vi "深国电程序控制(new).vi"(11 "槽位号":i16=1) -> ()   [LabVIEW 2012]
doc: "打开板卡操作，输出板卡句柄！当有多个板卡时，根据板卡索引号打开不同板卡！\n如果同时使用一块板卡的多种功能，可将输出句柄连接到不同的功能任务中。\n此VI是创建所有任务的前提！"
uses:
  P3060NEW/_SubVI/dll/P3060.dll
panel:
  in  "error IO":errorcluster
  out "波形图":i32[](graph)
  in  "read":bool caption="确定按钮"
  in  "LED¿ØÖÆû":bool
  in  "FPGA-Bit文件路径":path
  in  "加载程序":bool caption="确定按钮"
  in  "取消按钮":bool
  out "error out":errorcluster caption="错误警告"
  # "c"
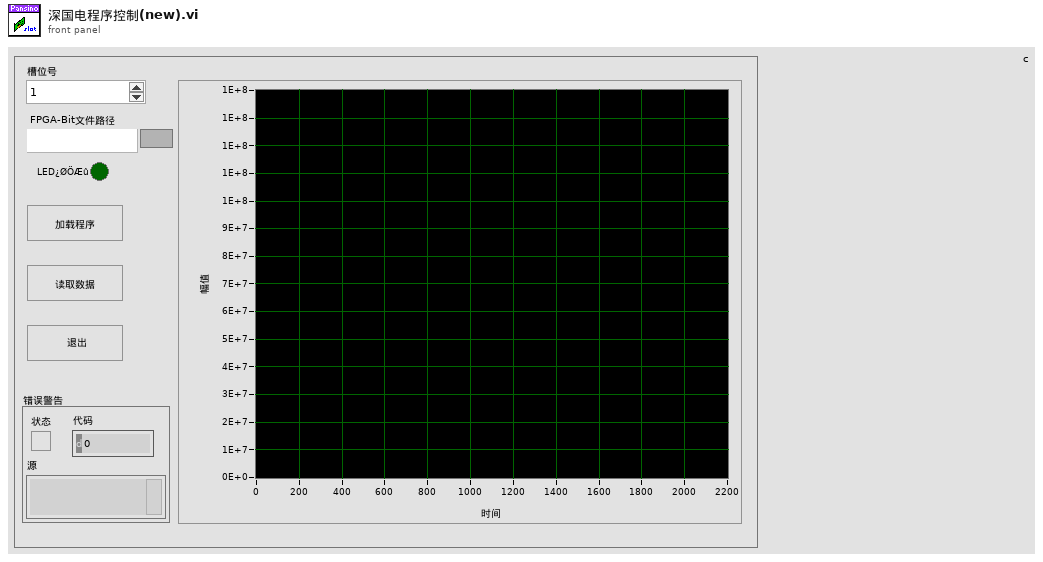
[diagram p1: front panel]
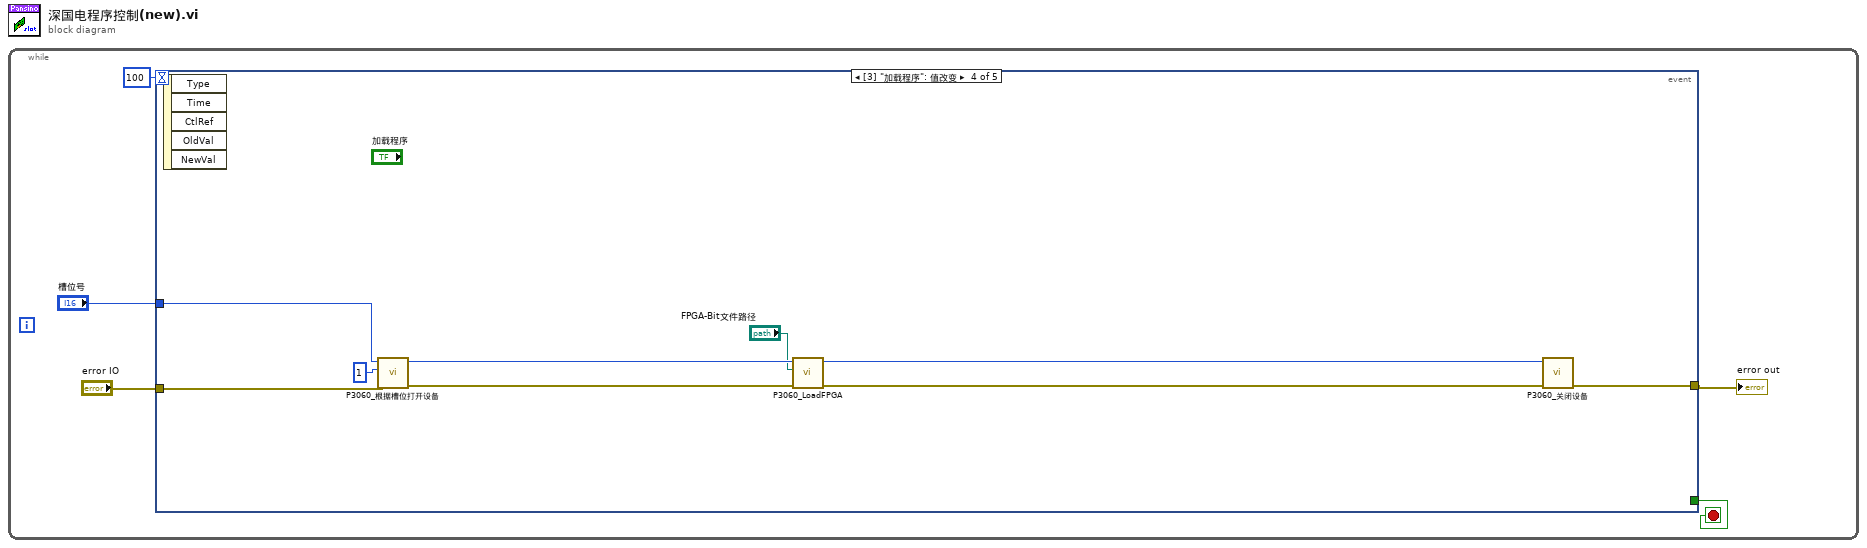
[diagram p0: block diagram]
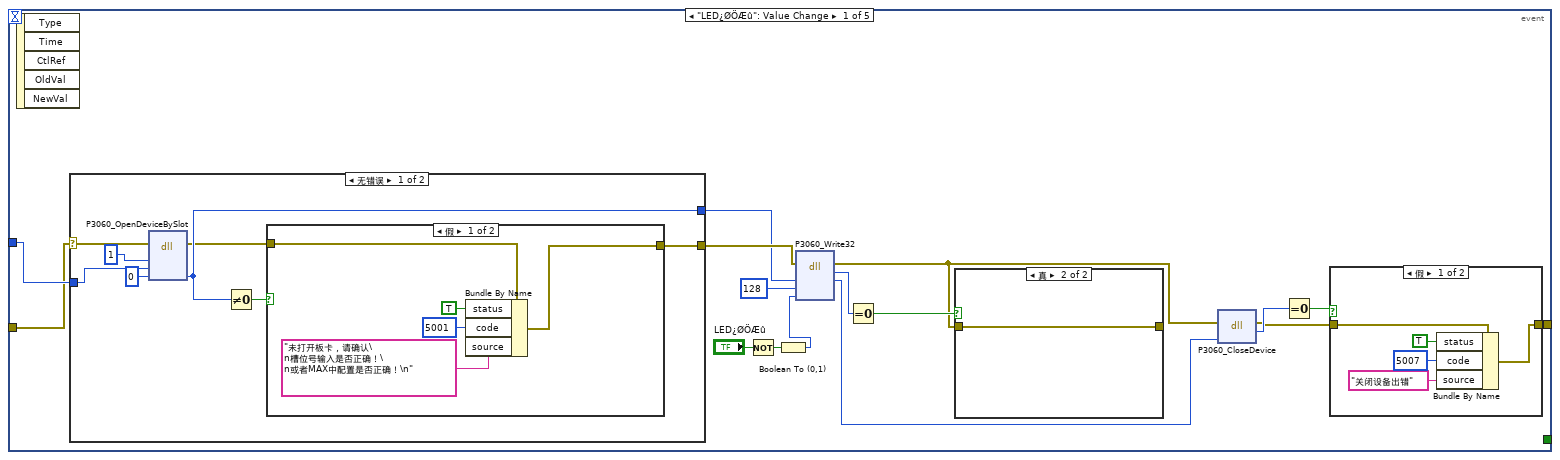
[diagram p2: hidden frame]
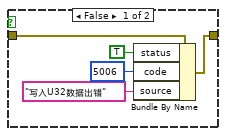
[diagram p3: hidden frame]
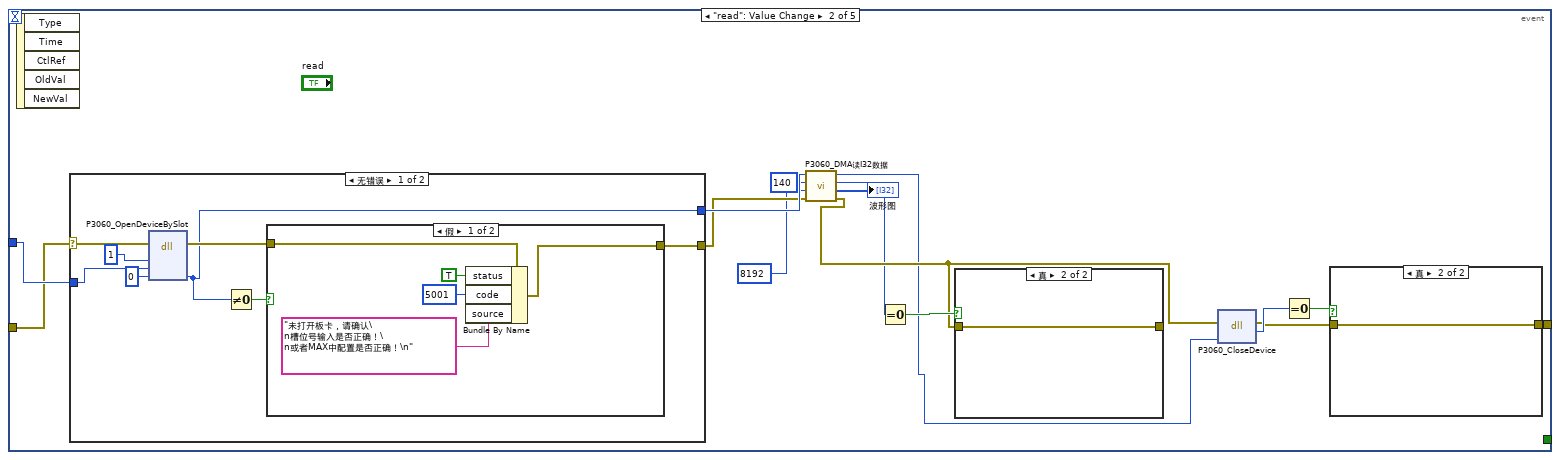
[diagram p7: hidden frame]
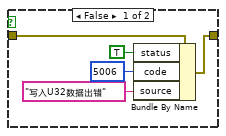
[diagram p8: hidden frame]
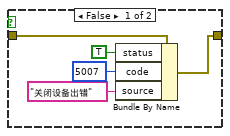
[diagram p9: hidden frame]
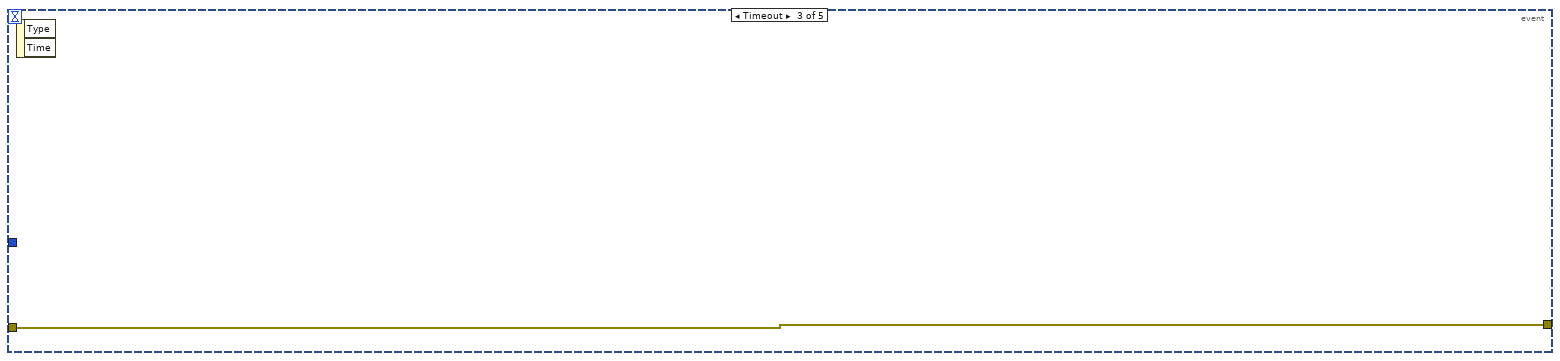
[diagram p12: hidden frame]
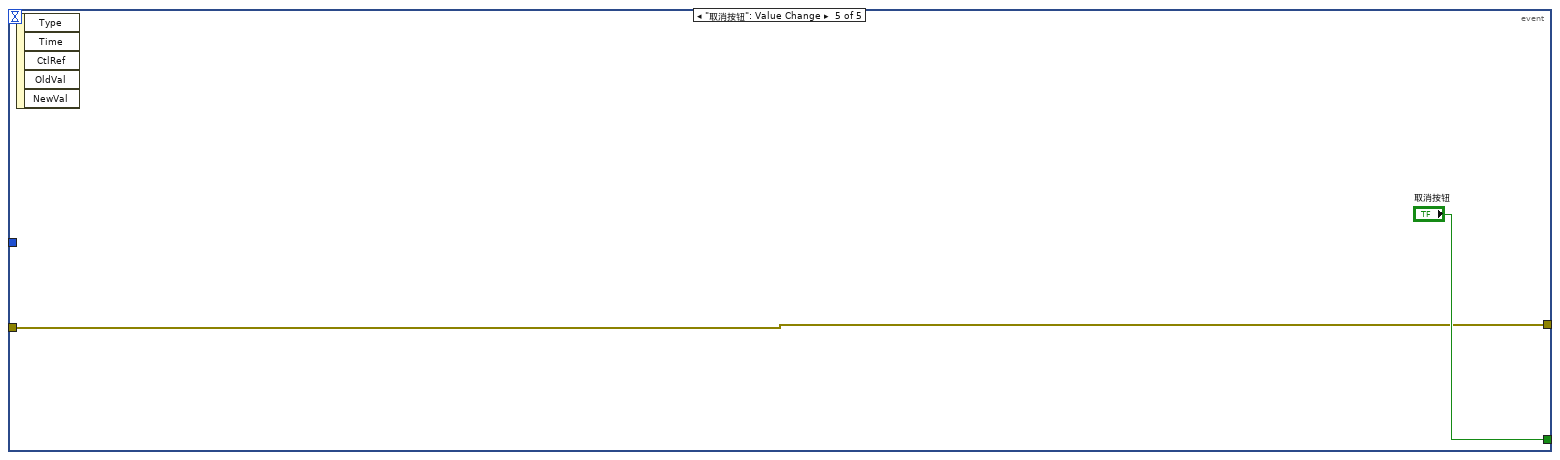
[diagram p13: hidden frame]
diagram:
  n1 = while {
    stop <- w5 stop-if-true
    n2 = event shown="[3] \"加载程序\": 值改变" {
      selector: _ -> [_ _ _ _ _]
      dyn-events: _ -> [_ _ _ _ _]
      timeout: 100 -> [_ _ _ _ _]
      tunnel: [_ _ _ _ "取消按钮"] -> w5
      tunnel: "槽位号" -> [w11 w50 _ w92 _]
      tunnel: [w9 w59 w91 w99 w101] -> w2
      tunnel: "error IO" -> [w10 w49 w91 w100 w101]
      event "LED¿ØÖÆû": Value Change {
        n3 = event-data() -> ()  [unwired: 1 in, 5 out]
        n4 = case shown="无错误" w10 {
          selector: w10 -> [w41 w48]
          tunnel: [w38 w48] -> w16
          tunnel: w11 -> [w40 _]
          tunnel: [w37 _] -> w14
          frame No Error {
            n5 = dll-call lib="C:/PLC_simulation/2014.3.9PLC_NEW/PLC_NEW/P3060NEW/_SubVI/dll/P3060.dll" fn="P3060_OpenDeviceBySlot"(error in=w41, "Classis"=i16 1, "槽位号"=w40, "设备句柄"=0) -> (error out=w34:errorcluster, "设备句柄"=w37:i32)  [unwired: 5 in, 1 out]
            n6 = Not Equal To 0?(x=w37) -> (x != 0?=w39:bool)
            n7 = case shown="假" w39 {
              tunnel: w34 -> [w46 w47]
              tunnel: [w42 w47] -> w38
              frame False {
                n8 = Bundle By Name(cluster=w46, "status"=TRUE, "code"=5001, "source"="未打开板卡，请确认\n槽位号输入是否正确！\n或者MAX中配置是否正确！\n") -> (w42:errorcluster)
              }
              frame True {
              }
            }
          }
          frame Error {
          }
        }
        n9 = Not(x="LED¿ØÖÆû") -> (.not. x?=w7:bool)
        n10 = Boolean To (0,1)(Boolean=w7) -> (0, 1=w8:i16)
        n11 = dll-call lib="C:/PLC_simulation/2014.3.9PLC_NEW/PLC_NEW/P3060NEW/_SubVI/dll/P3060.dll" fn="P3060_Write32"(error in=w16, "hDev"=w14, "Offset"=u32 128, "data"=w8) -> (error out=w15:errorcluster, "return"=w18:i32, "hDev"=w13:i32)  [unwired: 4 in, 1 out]
        n12 = Equal To 0?(x=w18) -> (x = 0?=w17:bool)
        n13 = case shown="真" w17 {
          tunnel: [w25 w27] -> _
          tunnel: w15 -> [w26 w27]
          frame False {
            n14 = Bundle By Name(cluster=w26, "status"=TRUE, "code"=5006, "source"="写入U32数据出错") -> (w25:errorcluster)
          }
          frame True {
          }
        }
        n15 = dll-call lib="C:/PLC_simulation/2014.3.9PLC_NEW/PLC_NEW/P3060NEW/_SubVI/dll/P3060.dll" fn="P3060_CloseDevice"(error in=w15, "hDev"=w13) -> (error out=w19:errorcluster, "hDevOut"=w21:i32)  [unwired: 3 in, 1 out]
        n16 = Equal To 0?(x=w21) -> (x = 0?=w20:bool)
        n17 = case shown="假" w20 {
          tunnel: [w31 w33] -> w9
          tunnel: w19 -> [w32 w33]
          frame False {
            n18 = Bundle By Name(cluster=w32, "status"=TRUE, "code"=5007, "source"="关闭设备出错") -> (w31:errorcluster)
          }
          frame True {
          }
        }
      }
      event "read": Value Change {
        n19 = event-data() -> ()  [unwired: 1 in, 5 out]
        n20 = case shown="无错误" w49 {
          selector: w49 -> [w83 w90]
          tunnel: [w79 w90] -> w57
          tunnel: w50 -> [w82 _]
          tunnel: [w76 _] -> w58
          frame No Error {
            n21 = dll-call lib="C:/PLC_simulation/2014.3.9PLC_NEW/PLC_NEW/P3060NEW/_SubVI/dll/P3060.dll" fn="P3060_OpenDeviceBySlot"(error in=w83, "Classis"=i16 1, "槽位号"=w82, "设备句柄"=0) -> (error out=w80:errorcluster, "设备句柄"=w76:i32)  [unwired: 5 in, 1 out]
            n22 = Not Equal To 0?(x=w76) -> (x != 0?=w81:bool)
            n23 = case shown="假" w81 {
              tunnel: w80 -> [w88 w89]
              tunnel: [w84 w89] -> w79
              frame False {
                n24 = Bundle By Name(cluster=w88, "status"=TRUE, "code"=5001, "source"="未打开板卡，请确认\n槽位号输入是否正确！\n或者MAX中配置是否正确！\n") -> (w84:errorcluster)
              }
              frame True {
              }
            }
          }
          frame Error {
          }
        }
        n25 = call "P3060_DMA读I32数据.vi"("错误输入"=w57, "数据长度"=u32 8192, "偏移地址"=u32 140, "句柄输入"=w58) -> ("错误输出"=w56:errorcluster, "读I32数据"=→"波形图":i32[], "返回值"=w55:i32, "句柄输出"=w54:i32)  [unwired: 4 in]
        n26 = Equal To 0?(x=w55) -> (x = 0?=w60:bool)
        n27 = case shown="真" w60 {
          tunnel: [w67 w69] -> _
          tunnel: w56 -> [w68 w69]
          frame False {
            n28 = Bundle By Name(cluster=w68, "status"=TRUE, "code"=5006, "source"="写入U32数据出错") -> (w67:errorcluster)
          }
          frame True {
          }
        }
        n29 = dll-call lib="C:/PLC_simulation/2014.3.9PLC_NEW/PLC_NEW/P3060NEW/_SubVI/dll/P3060.dll" fn="P3060_CloseDevice"(error in=w56, "hDev"=w54) -> (error out=w61:errorcluster, "hDevOut"=w63:i32)  [unwired: 3 in, 1 out]
        n30 = Equal To 0?(x=w63) -> (x = 0?=w62:bool)
        n31 = case shown="真" w62 {
          tunnel: [w73 w75] -> w59
          tunnel: w61 -> [w74 w75]
          frame False {
            n32 = Bundle By Name(cluster=w74, "status"=TRUE, "code"=5007, "source"="关闭设备出错") -> (w73:errorcluster)
          }
          frame True {
          }
        }
      }
      event Timeout {
        n33 = event-data() -> ()  [unwired: 1 in, 2 out]
      }
      event "加载程序": Value Change {
        n34 = event-data() -> ()  [unwired: 1 in, 5 out]
        n35 = call "P3060_根据槽位打开设备.vi"("error in (no error)"=w100, "机箱号"=i16 1, "槽位号"=w92) -> ("error out"=w96:errorcluster, "句柄输出"=w94:i32)  [unwired: 7 in]
        n36 = call "P3060_LoadFPGA.vi"("错误输入"=w96, "Bit文件路径"="FPGA-Bit文件路径", "句柄输入"=w94) -> ("错误输出"=w98:errorcluster, "句柄输出"=w97:i32)  [unwired: 6 in, 1 out]
        n37 = call "P3060_关闭设备.vi"("error in (no error)"=w98, "句柄输入"=w97) -> ("error out"=w99:errorcluster)  [unwired: 9 in]
      }
      event "取消按钮": Value Change {
        n38 = event-data() -> ()  [unwired: 1 in, 5 out]
      }
    }
    "error out" <- w2
  }
